vi "MQTT_Q_Connect.vi"(7 "Connect Flags and Keep Alive":T4={"user name"=FALSE, "password"=FALSE, "will retain"=FALSE, "will QoS"=enum."At most once", "will flag"=FALSE, "clean session"=TRUE, "reserved"=FALSE, "Keep Alive (sec)"=60}, 8 "error in (no error)":errorcluster, 9 "User and Will Parameters":T2, 11 "MQTT Broker & Client ID":T1={"IP address"="localhost", "Port"=1883, "Client ID"=""}) -> (0 "error out":errorcluster, 3 "MQTT_Q Out":refnum<class "MQTT_Q.lvclass">)   [LabVIEW 2015, in "MQTT_Q.lvclass"]
uses:
  MQTT_Q.lvclass
  MQTT_Q_QoS.ctl
  MQTT_Q_PVT_MessageType.ctl
  MQTT_Q.lvclass/MQTT_Q.ctl
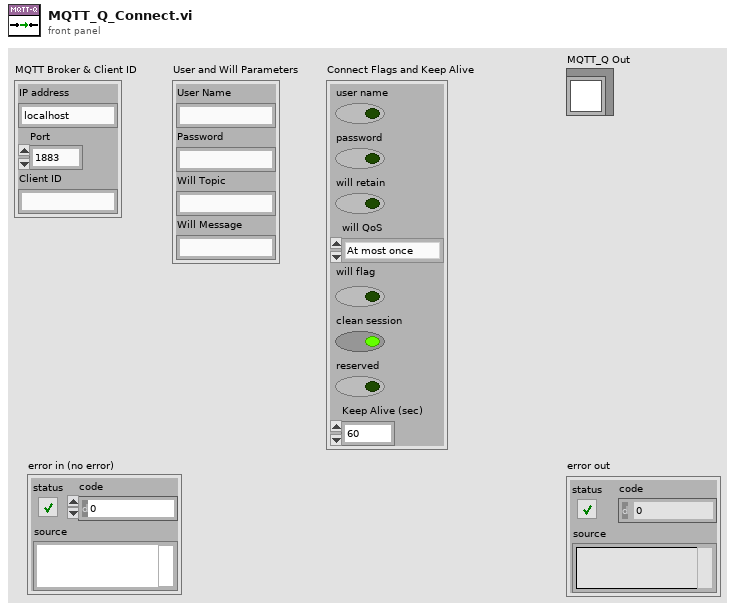
[diagram p1: front panel]
types:
  T1 = cluster{"IP address":string, "Port":u16, "Client ID":string}
  T2 = cluster{"User Name":string, "Password":string, "Will Topic":string, "Will Message":string}
  T3 = typedef "MQTT_Q.lvclass/MQTT_Q_QoS.ctl" = enum8{"At most once", "At least once", "Exactly once", "Reserved"}
  T4 = cluster{"user name":bool, "password":bool, "will retain":bool, "will QoS":T3, "will flag":bool, "clean session":bool, "reserved":bool, "Keep Alive (sec)":u16}
  T5 = typedef "MQTT_Q.lvclass/MQTT_Q_PVT_MessageType.ctl" = enum32{"Reserved", "CONNECT", "CONNACK", "PUBLISH", "PUBACK", "PUBREC", "PUBREL", "PUBCOMP", "SUBSCRIBE", "SUBACK", "UNSUBSCRIBE", "UNSUBACK", "PINGREQ", "PINGRESP", "DISCONNECT", "Reserved2"}
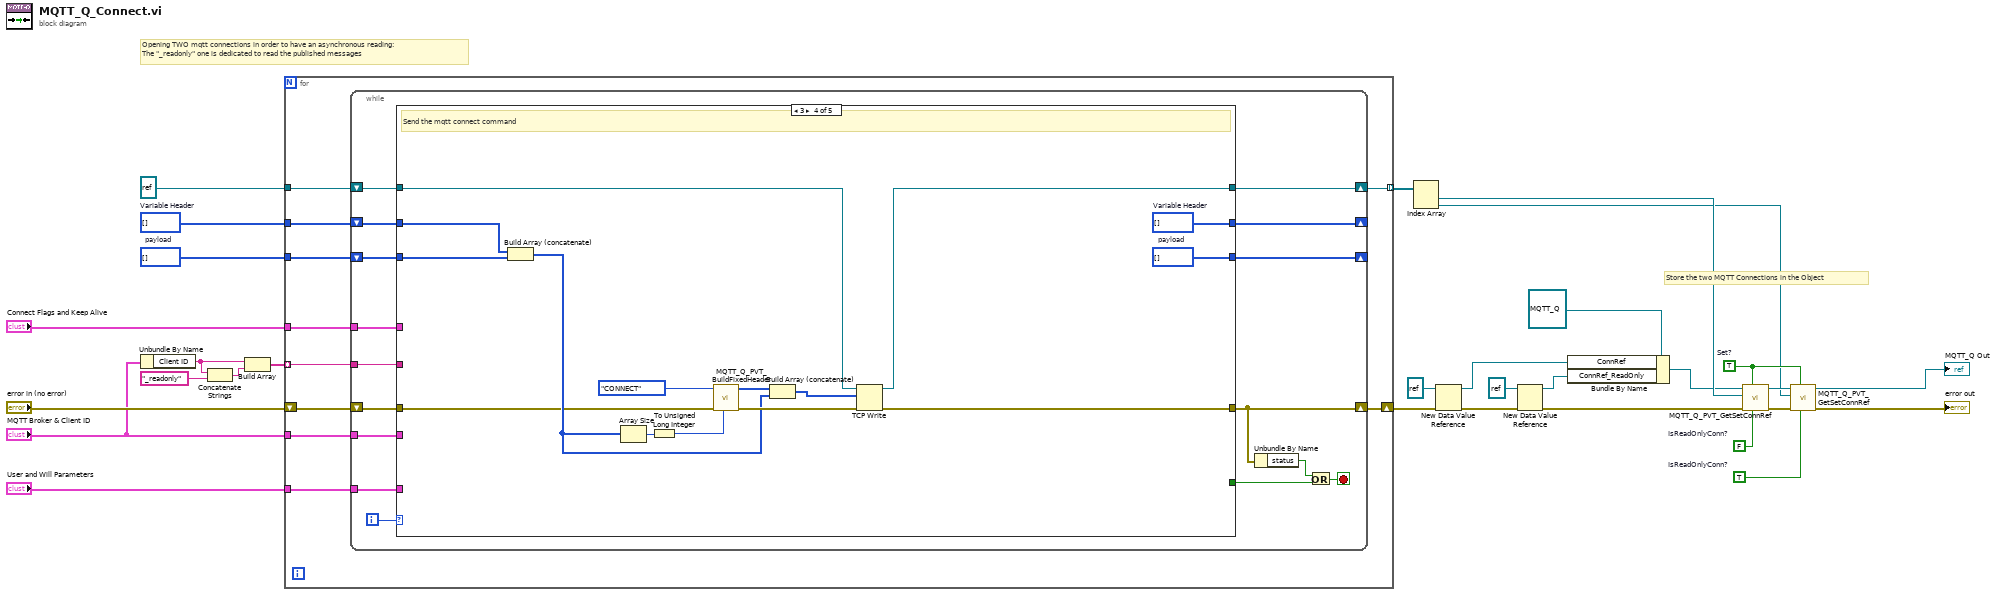
[diagram p0: block diagram]
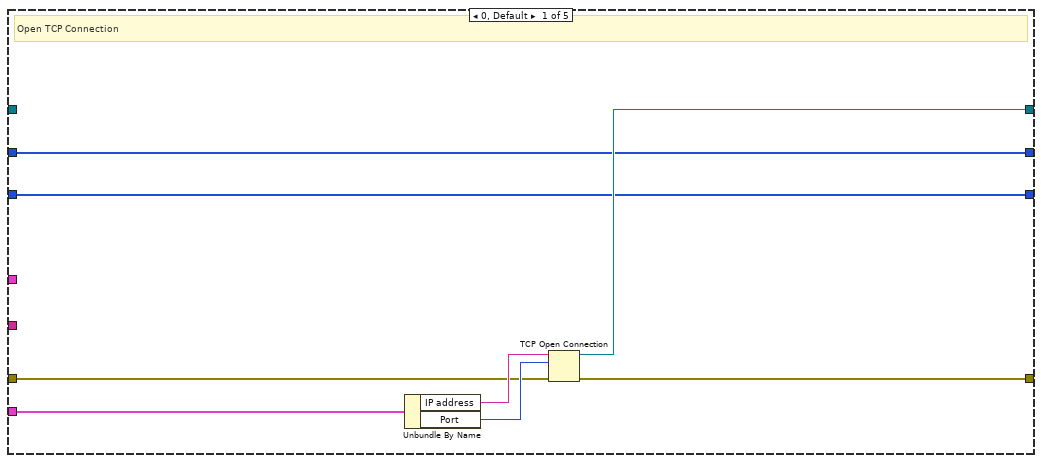
[diagram p2: hidden frame]
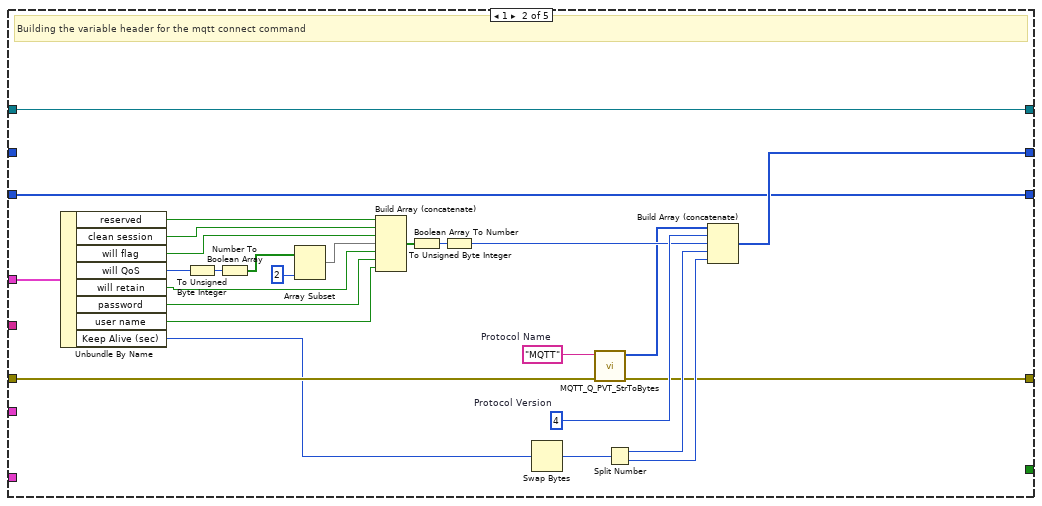
[diagram p3: hidden frame]
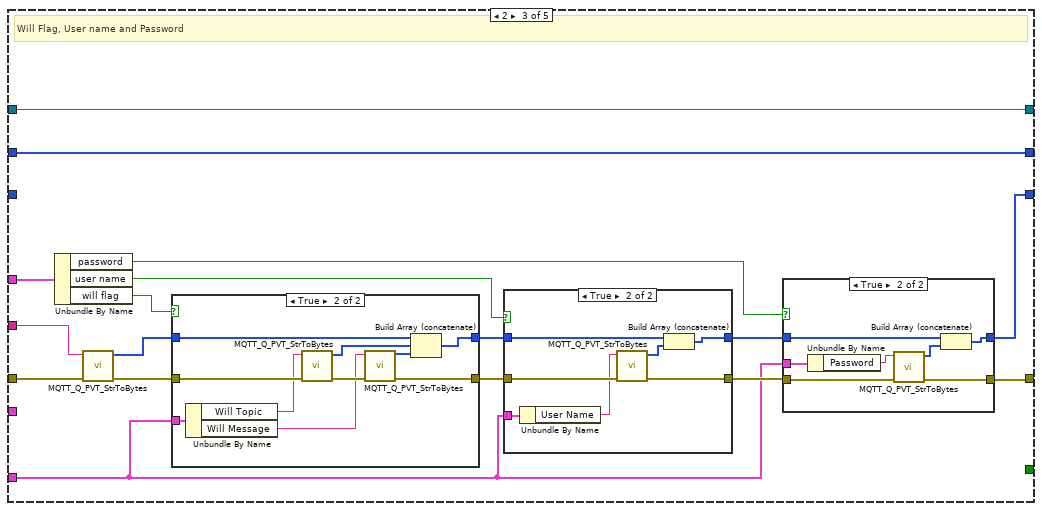
[diagram p4: hidden frame]
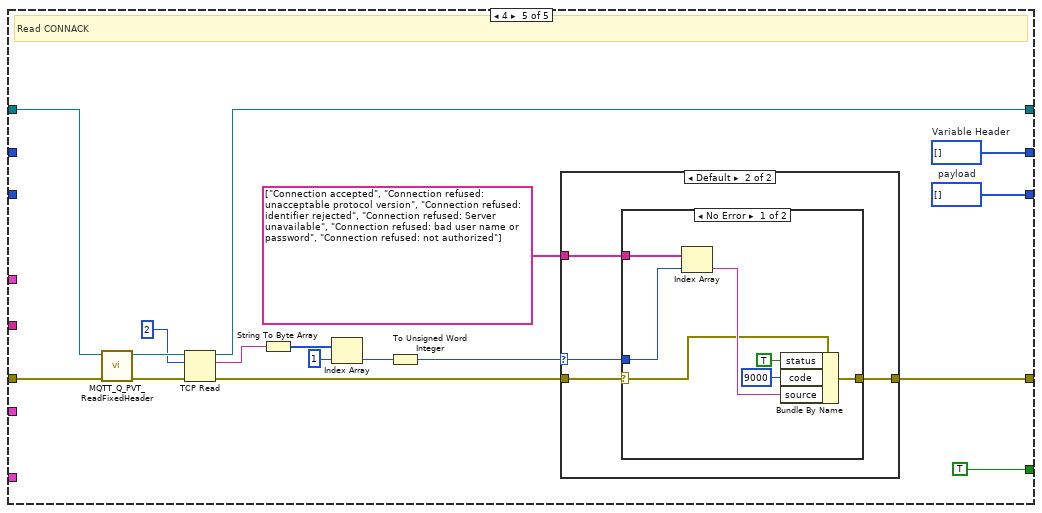
[diagram p8: hidden frame]
diagram:
  w13 = FALSE  # IsReadOnlyConn?
  w14 = TRUE  # IsReadOnlyConn?
  w16 = TRUE  # Set?
  w26 = u8[] []  # payload
  w27 = u8[] []  # Variable Header
  # "Store the two MQTT Connections in the Object"
  # "Opening TWO mqtt connections in order to have an asynchronous reading:\nThe \"_readonly\" one is dedicated to read the published messages"
  n1 = Unbundle By Name("MQTT Broker & Client ID") -> ("Client ID"=w1:string)
  n2 = Concatenate Strings(w1, "_readonly" ("string")) -> (w22:string)
  n3 = Build Array(w1, w22) -> (w21:string[])
  n4 = for {
    tunnel: "MQTT Broker & Client ID" -> [w39]
    tunnel: w21 -> [w38] mode=indexing
    tunnel: "Connect Flags and Keep Alive" -> [w37]
    tunnel: w27 -> [w35]
    tunnel: w26 -> [w34]
    shift-right: [w33] -> w5
    shift-left: "error in (no error)" -> [w40]
    tunnel: refnum<k5> refnum ("connection ID out") -> [w36]
    tunnel: [w32] -> w24 mode=indexing
    tunnel: "User and Will Parameters" -> [w31]
    n5 = while {
      shift-right: [w45] -> w33
      shift-left: w40 -> [w54]
      tunnel: w39 -> [w55]
      shift-right: [w53] -> w32
      shift-left: w36 -> [w50]
      tunnel: w38 -> [w52]
      tunnel: w37 -> [w51]
      shift-right: [w49] -> _
      shift-left: w35 -> [w47]
      shift-right: [w48] -> _
      shift-left: w34 -> [w46]
      tunnel: w31 -> [w41]
      i -> [w56]
      stop <- w43 stop-if-true
      n6 = case shown="3" w56 {
        tunnel: w55 -> [w62 _ _ _ _]
        tunnel: w54 -> [w61 w86 w99 w146 w169]
        tunnel: [w60 w85 w97 w140 w164] -> w45
        tunnel: [w59 w91 w100 w139 w167] -> w53
        tunnel: w52 -> [_ _ w94 _ _]
        tunnel: w51 -> [_ w71 w101 _ _]
        tunnel: w50 -> [_ w91 w100 w145 w168]
        tunnel: [w58 w69 w95 w144 w166] -> w49
        tunnel: [w57 w68 w96 w143 w165] -> w48
        tunnel: w47 -> [w58 _ w95 w142 _]
        tunnel: w46 -> [w57 w68 _ w141 _]
        tunnel: [_ _ _ _ TRUE] -> w42
        tunnel: w41 -> [_ _ w92 _ _]
        frame 0, Default {
          # "Open TCP Connection"
          n7 = Unbundle By Name(w62) -> ("IP address"=w63:string, "Port"=w64:u16)
          n8 = TCP Open Connection(address=w63, remote port or service name=w64, error in (no error)=w61) -> (connection ID=w59:refnum<k5>, error out=w60:errorcluster)  [unwired: 2 in]
        }
        frame 1 {
          w87 = u8 4  # Protocol Version
          w67 = "MQTT"  # Protocol Name
          # "Building the variable header for the mqtt connect command"
          n9 = Unbundle By Name(w71) -> ("reserved"=w75:bool, "clean session"=w76:bool, "will flag"=w77:bool, "will QoS"=w79:T3, "will retain"=w82:bool, "password"=w81:bool, "user name"=w80:bool, "Keep Alive (sec)"=w65:u16)
          n10 = To Unsigned Byte Integer(number=w79) -> (unsigned 8bit integer=w72:u8)
          n11 = Number To Boolean Array(number=w72) -> (Boolean array=w73:bool[])
          n12 = Array Subset(array=w73, length=2) -> (w78:bool[])  [unwired: 1 in]
          n13 = Build Array (concatenate)(w75, w76, w77, w78, w82, w81, w80) -> (w83:bool[])
          n14 = Boolean Array To Number(Boolean array=w83) -> (number=w84:u32)
          n15 = To Unsigned Byte Integer(number=w84) -> (unsigned 8bit integer=w70:u8)
          n16 = Swap Bytes(anything=w65) -> (byte swapped=w90:u16)
          n17 = call "MQTT_Q_PVT_StrToBytes.vi"("error in (no error)"=w86, "String in"=w67) -> ("error out"=w85:errorcluster, "Bytes out"=w66:u8[])  [unwired: 8 in]
          n18 = Split Number(x=w90) -> (hi(x)=w89:u8, lo(x)=w88:u8)
          n19 = Build Array (concatenate)(w66, w87, w70, w89, w88) -> (w69:u8[])
        }
        frame 2 {
          # "Will Flag, User name and Password"
          n20 = Unbundle By Name(w101) -> ("password"=w104:bool, "user name"=w107:bool, "will flag"=w108:bool)
          n21 = call "MQTT_Q_PVT_StrToBytes.vi"("error in (no error)"=w99, "String in"=w94) -> ("error out"=w98:errorcluster, "Bytes out"=w93:u8[])  [unwired: 8 in]
          n22 = case shown="True" w108 {
            tunnel: w93 -> [w128 w137]
            tunnel: [w128 w138] -> w102
            tunnel: w98 -> [w127 w136]
            tunnel: [w127 w134] -> w106
            tunnel: w92 -> [_ w133]
            frame False {
            }
            frame True {
              n23 = Unbundle By Name(w133) -> ("Will Topic"=w132:string, "Will Message"=w131:string)
              n24 = call "MQTT_Q_PVT_StrToBytes.vi"("error in (no error)"=w136, "String in"=w132) -> ("error out"=w135:errorcluster, "Bytes out"=w130:u8[])  [unwired: 8 in]
              n25 = call "MQTT_Q_PVT_StrToBytes.vi"("error in (no error)"=w135, "String in"=w131) -> ("error out"=w134:errorcluster, "Bytes out"=w129:u8[])  [unwired: 8 in]
              n26 = Build Array (concatenate)(w137, w130, w129) -> (w138:u8[])
            }
          }
          n27 = case shown="True" w107 {
            tunnel: w102 -> [w119 w126]
            tunnel: [w119 w125] -> w103
            tunnel: [w118 w124] -> w105
            tunnel: w106 -> [w118 w123]
            tunnel: w92 -> [_ w122]
            frame False {
            }
            frame True {
              n28 = Unbundle By Name(w122) -> ("User Name"=w121:string)
              n29 = call "MQTT_Q_PVT_StrToBytes.vi"("error in (no error)"=w123, "String in"=w121) -> ("error out"=w124:errorcluster, "Bytes out"=w120:u8[])  [unwired: 8 in]
              n30 = Build Array (concatenate)(w126, w120) -> (w125:u8[])
            }
          }
          n31 = case shown="True" w104 {
            tunnel: w103 -> [w110 w117]
            tunnel: [w110 w116] -> w96
            tunnel: w105 -> [w109 w115]
            tunnel: [w109 w114] -> w97
            tunnel: w92 -> [_ w113]
            frame False {
            }
            frame True {
              n32 = Unbundle By Name(w113) -> ("Password"=w111:string)
              n33 = call "MQTT_Q_PVT_StrToBytes.vi"("error in (no error)"=w115, "String in"=w111) -> ("error out"=w114:errorcluster, "Bytes out"=w112:u8[])  [unwired: 8 in]
              n34 = Build Array (concatenate)(w117, w112) -> (w116:u8[])
            }
          }
        }
        frame 3 {
          w143 = u8[] []  # payload
          w144 = u8[] []  # Variable Header
          # "Send the mqtt connect command"
          n35 = Build Array (concatenate)(w142, w141) -> (w148:u8[])
          n36 = Array Size(array=w148) -> (size(s)=w150:i32)
          n37 = To Unsigned Long Integer(number=w150) -> (unsigned 32bit integer=w151:u32)
          n38 = call "MQTT_Q_PVT_BuildFixedHeader.vi"("Remaining Length"=w151, "error in (no error)"=w146, "MessageType"=MQTT_Q_PVT_MessageType."CONNECT") -> ("error out"=w152:errorcluster, "Fixed Header"=w149:u8[])  [unwired: 7 in]
          n39 = Build Array (concatenate)(w149, w148) -> (w153:u8[])
          n40 = TCP Write(connection ID=w145, data in=w153, error in (no error)=w152) -> (connection ID out=w139:refnum<k5>, error out=w140:errorcluster)  [unwired: 1 in, 1 out]
        }
        frame 4 {
          w165 = u8[] []  # payload
          w166 = u8[] []  # Variable Header
          # "Read CONNACK"
          n41 = call "MQTT_Q_PVT_ReadFixedHeader.vi"("error in"=w169, "connection ID"=w168) -> ("error out"=w160:errorcluster, "connection ID out"=w161:refnum<k5>)  [unwired: 6 in, 2 out]
          n42 = TCP Read(connection ID=w161, bytes to read=2, error in (no error)=w160) -> (connection ID out=w167:refnum<k5>, data out=w158:string, error out=w156:errorcluster)  [unwired: 2 in]
          n43 = String To Byte Array(string=w158) -> (unsigned byte array=w157:u8[])
          n44 = Index Array(array=w157, index=1) -> (element=w163:u8)
          n45 = To Unsigned Word Integer(number=w163) -> (unsigned 16bit integer=w155:u16)
          n46 = case shown="Default" w155 {
            selector: w155 -> [_ w173]
            tunnel: w156 -> [w171 w175]
            tunnel: [w171 w174] -> w164
            tunnel: string[] ["Connection accepted", "Connection refused: unacceptable protocol version", "Connection refused: identifier rejected", "Connection refused: Server unavailable", "Connection refused: bad user name or password", "Connection refused: not authorized"] ("Strings []") -> [_ w172]
            frame 0 {
              # "0 = Connection Accepted"
            }
            frame Default {
              n47 = case shown="No Error" w175 {
                selector: w175 -> [w177 w183]
                tunnel: [w182 w183] -> w174
                tunnel: w173 -> [w179 _]
                tunnel: w172 -> [w180 _]
                frame No Error {
                  n48 = Index Array(array=w180, index=w179) -> (element=w178:string)
                  n49 = Bundle By Name(cluster=w177, "status"=TRUE, "code"=9000, "source"=w178) -> (w182:errorcluster)
                }
                frame Error {
                }
              }
            }
          }
        }
      }
      n50 = Unbundle By Name(w45) -> ("status"=w44:bool)
      n51 = Or(x=w44, y=w42) -> (x .or. y?=w43:bool)
    }
  }
  n52 = Index Array(array=w24) -> (element #1=w25:refnum<k5>, element #2=w15:refnum<k5>)  [unwired: 2 in]
  n53 = New Data Value Reference(data value=refnum<k5> refnum ("connection ID out"), error in=w5) -> (data value reference=w10:refnum<data-value>, error out=w8:errorcluster)
  n54 = New Data Value Reference(data value=refnum<k5> refnum ("connection ID out"), error in=w8) -> (data value reference=w7:refnum<data-value>, error out=w4:errorcluster)
  n55 = Bundle By Name(cluster=refnum<class "MQTT_Q.lvclass"> refnum ("MQTT_Q In"), "ConnRef"=w10, "ConnRef_ReadOnly"=w7) -> (w3:refnum<class "MQTT_Q.lvclass">)
  n56 = call "MQTT_Q_PVT_GetSetConnRef.vi"("IsReadOnlyConn?"=w13, "Set?"=w16, "error in (no error)"=w4, "connection ID In"=w25, "MQTT_Q in"=w3) -> ("error out"=w18:errorcluster, "MQTT_Q out"=w20:refnum<class "MQTT_Q.lvclass">)  [unwired: 4 in, 1 out]
  n57 = call "MQTT_Q_PVT_GetSetConnRef.vi"("IsReadOnlyConn?"=w14, "Set?"=w16, "error in (no error)"=w18, "connection ID In"=w15, "MQTT_Q in"=w20) -> ("error out"=→"error out":errorcluster, "MQTT_Q out"=→"MQTT_Q Out":refnum<class "MQTT_Q.lvclass">)  [unwired: 4 in, 1 out]
